vi "GetCompass.vi"(11 "Compass In":refnum<visa-resource-name>) -> (0 "compassHeading":dbl format="%#.3g", 3 "Compass Out":refnum<visa-resource-name>)   [LabVIEW 2011]
uses:
  <instrlib>/Ocean Server OS4000/Ocean Server OS4000.lvlib
panel:
  out "rollAngle":dbl format="%#.3g"
  out "pitchAngle":dbl format="%#.3g"
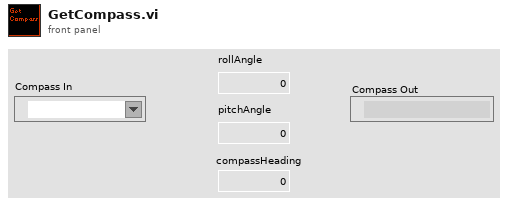
[diagram p1: front panel]
types:
  T1 = cluster{"Compass Heading":dbl, "pitch Angle":dbl, "roll Angle":dbl, "Temperature":dbl, "Depth":dbl, "Magnetic Field":dbl, "Magnetic Field X":dbl, "Magnetic Field Y":dbl, "Magnetic Field Z":dbl, "Acceleration":dbl, "Acceleration X":dbl, "Acceleration Y":dbl, "Gyro":dbl, "Gyro X":dbl, "Acceleration Z":dbl, "Gyro Y":dbl}
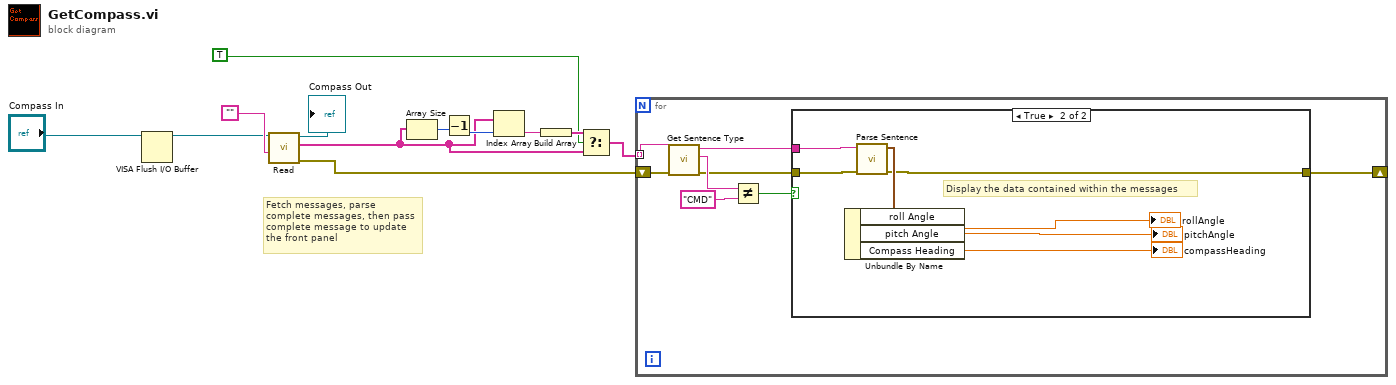
[diagram p0: block diagram]
diagram:
  # "Fetch messages, parse complete messages, then pass  complete message to update the front panel"
  n1 = VISA Flush I/O Buffer(VISA resource name="Compass In") -> (VISA resource name out=w2:refnum<visa-resource-name>)  [unwired: 2 in, 1 out]
  n2 = call <instrlib>:"Read.vi"("Text to prepend to sentence"="" ("Remaining String"), "VISA resource name"=w2) -> ("error out"=w11:errorcluster, "Ocean Server Sentences"=w6:string[], "VISA resource name out"=→"Compass Out":refnum<visa-resource-name>)  [unwired: 6 in, 1 out]
  n3 = Array Size(array=w6) -> (size(s)=w10:i32)
  n4 = Decrement(x=w10) -> (x-1=w9:i32)
  n5 = Index Array(array=w6, index=w9) -> (element=w8:string)
  n6 = Build Array(w8) -> (w7:string[])
  n7 = Select(t=w7, s=TRUE, f=w6) -> (s? t:f=w5:string[])
  n8 = for {
    tunnel: w5 -> [w20] mode=indexing
    shift-right: [w13] -> _
    shift-left: w11 -> [w14]
    n9 = call <instrlib>:"Get Sentence Type.vi"("error in (no error)"=w14, "Sentence In"=w20) -> ("error out"=w15:errorcluster, "Sentence Type"=w19:string, "Sentence Out"=w16:string)  [unwired: 7 in]
    n10 = Not Equal?(x=w19, y="CMD") -> (x != y?=w17:bool)
    n11 = case shown="True" w17 {
      tunnel: w16 -> [_ w25]
      tunnel: w15 -> [w21 w22]
      tunnel: [w21 w23] -> w13
      frame False {
        # "Front Panel isn't updated if the message received is not of the N1 type"
      }
      frame True {
        # "Display the data contained within the messages"
        n12 = call <instrlib>:"Parse Sentence.vi"("error in (no error)"=w22, "Ocean Server Sentence"=w25) -> ("error out"=w23:errorcluster, "Values"=w24:T1)  [unwired: 8 in]
        n13 = Unbundle By Name(w24) -> ("roll Angle"=→"rollAngle":dbl, "pitch Angle"=→"pitchAngle":dbl, "Compass Heading"=→"compassHeading":dbl)
      }
    }
  }
